vi "Start Aquisition.vi"(8 "error in (no error)":errorcluster, 10 "Buffer size":i64, 11 "HRF_Device":refnum<class "HRF_Device.lvclass">) -> (0 "error out":errorcluster, 3 "HRF_Device":refnum<class "HRF_Device.lvclass">)   [LabVIEW 2020, in "HRF_Device.lvclass"]
uses:
  HRF_Device.lvclass
  HRF_Device.lvclass/HRF_Device.ctl
  D:/work/HackRF/Labview Driver/NetHackrf.dll
  NetHackrf.dll
  Acquisition Daemon.vi
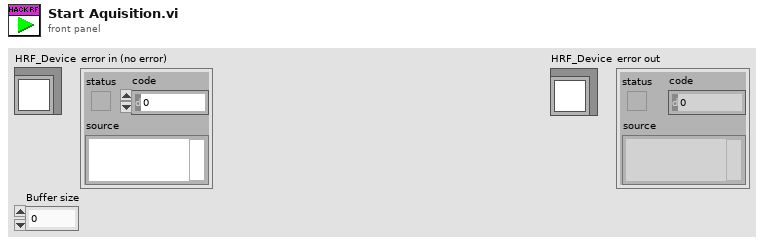
[diagram p1: front panel]
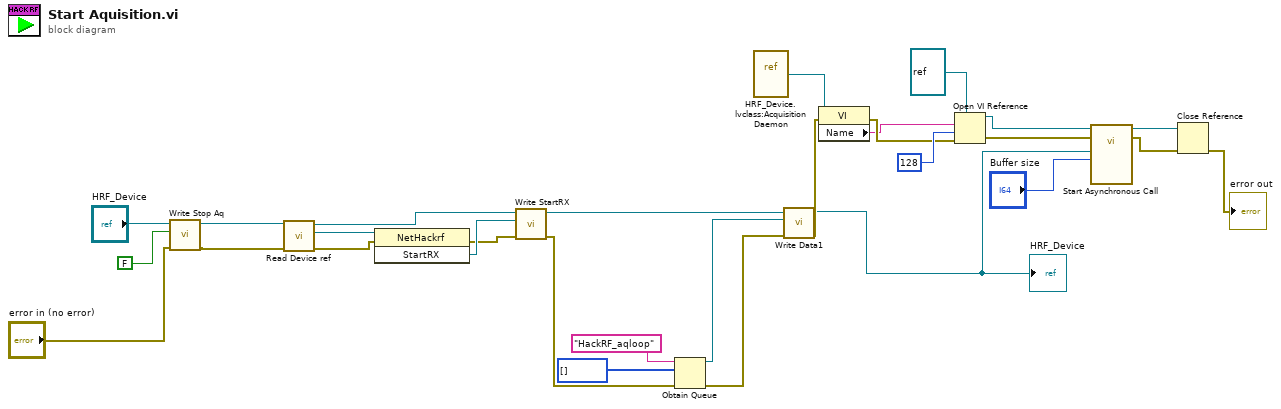
[diagram p0: block diagram]
diagram:
  n1 = call "Write Stop Aq.vi"("error in (no error)"="error in (no error)", "Stop Aq"=FALSE, "HRF_Device in"="HRF_Device") -> ("error out"=w12:errorcluster, "HRF_Device out"=w14:refnum<class "HRF_Device.lvclass">)  [unwired: 7 in]
  n2 = call "Read Device ref.vi"("error in (no error)"=w12, "HRF_Device in"=w14) -> ("error out"=w28:errorcluster, "Device ref"=w29:refnum<k24>, "HRF_Device out"=w27:refnum<class "HRF_Device.lvclass">)  [unwired: 7 in]
  n3 = invoke class="NetHackrf" method="StartRX"(reference=w29, error in=w28) -> (error out=w3:errorcluster, "StartRX"=w26:refnum<k24>)  [unwired: 1 in, 1 out]
  n4 = call "Write StartRX.vi"("error in (no error)"=w3, "StartRX"=w26, "HRF_Device in"=w27) -> ("error out"=w2:errorcluster, "HRF_Device out"=w8:refnum<class "HRF_Device.lvclass">)  [unwired: 7 in]
  n5 = Obtain Queue(name (unnamed)="HackRF_aqloop", element data type=i32[] [], error in (no error)=w2) -> (queue out=w6:refnum<queue>, error out=w7:errorcluster)  [unwired: 2 in, 1 out]
  n6 = vi-ref "HRF_Device.lvclass:Acquisition Daemon.vi"() -> (w18:refnum<vi>)
  n7 = call "Write Data1.vi"("error in (no error)"=w7, "Data"=w6, "HRF_Device in"=w8) -> ("error out"=w5:errorcluster, "HRF_Device out"=w1:refnum<class "HRF_Device.lvclass">)  [unwired: 7 in]
  "HRF_Device" <- w1
  n8 = property class="VI"(reference=w18, error in=w5) -> (error out=w20:errorcluster, "Name"=w19:string)  [unwired: 1 out]
  n9 = Open VI Reference(type specifier VI Refnum (for type only)=refnum<vi> refnum, vi path=w19, options=128, error in (no error)=w20) -> (vi reference=w23:refnum<vi>, error out=w22:errorcluster)  [unwired: 2 in]
  n10 = call-by-ref "Start Asynchronous Call"(reference=w23, error in=w22, "Buffer size"="Buffer size", "HRF_Device"=w1) -> (reference out=w17:refnum<vi>, error out=w16:errorcluster)  [unwired: 10 in]
  n11 = Close Reference(reference=w17, error in (no error)=w16) -> (error out=→"error out":errorcluster)
